vi "actuate.vi"(0 "SingleCylinderActuator in":refnum<class "SingleCylinderActuator.lvclass">, 5 "ILC in":refnum<class "ILC.lvclass">, 7 "Actuate Settings":T1, 11 "error in (no error)":errorcluster) -> (4 "SingleCylinderActuator out":refnum<class "SingleCylinderActuator.lvclass">, 6 "ILC out":refnum<class "ILC.lvclass">, 15 "error out":errorcluster)   [LabVIEW 2015, in "SingleCylinderActuator.lvclass"]
uses:
  SingleCylinderActuator.lvclass
  <userlib>/Common/ILC/ILC/ILC.lvclass
  Typedefs/Actuate Settings.ctl
  Typedefs/ControlMode.ctl
  SingleCylinderActuator.lvclass/SingleCylinderActuator.ctl
  ActuatorCylinder/IActuatorCylinder/IActuatorCylinder.lvclass
  Calculators/ForceToPressureServoVoltage/ForceToPressureServoVoltage.lvclass
  Typedefs/FAMTTypedefs.lvlib
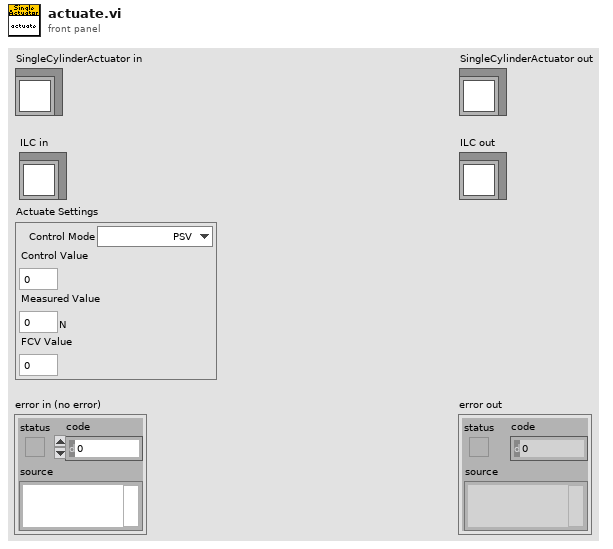
[diagram p1: front panel]
types:
  T1 = typedef "FAMTTypedefs.lvlib/Actuate Settings.ctl" = cluster{"Control Mode":T2, "Control Value":dbl, "Measured Value":dbl[unit], "FCV Value":dbl}
  T2 = typedef "FAMTTypedefs.lvlib/ControlMode.ctl" = enum16{"PSV", "FCV", "Both"}
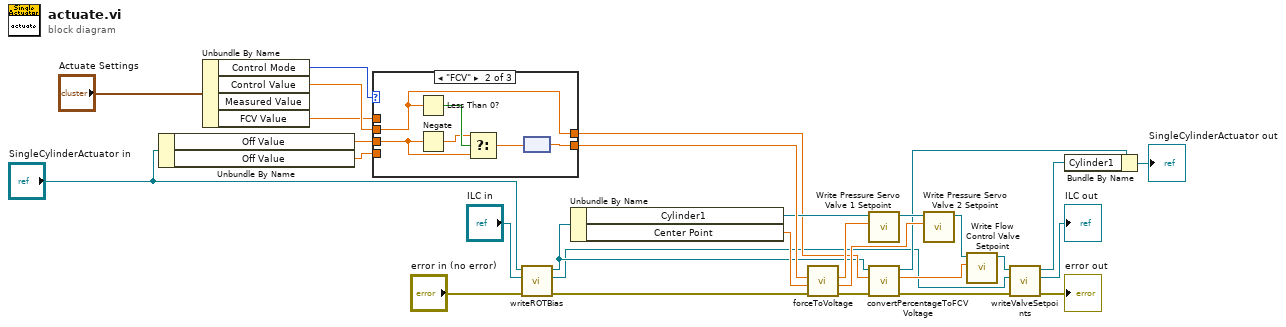
[diagram p0: block diagram]
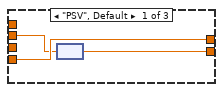
[diagram p2: hidden frame]
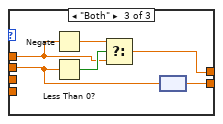
[diagram p3: hidden frame]
diagram:
  n1 = Unbundle By Name("SingleCylinderActuator in") -> ("Off Value"=w20:dbl, "Off Value"=w19:dbl)
  n2 = Unbundle By Name("Actuate Settings") -> ("Control Mode"=w25:T2, "Control Value"=w22:dbl, "FCV Value"=w21:dbl)  [unwired: 1 out]
  n3 = case shown="\"FCV\"" w25 {
    tunnel: w22 -> [w31 w37 w40]
    tunnel: w21 -> [_ _ w42]
    tunnel: w20 -> [_ w33 _]
    tunnel: w19 -> [w32 _ _]
    tunnel: [w32 w37 w41] -> w4
    tunnel: [w30 w38 w39] -> w18
    frame "PSV", Default {
      n4 = node(w31) -> (w30:dbl[unit])
    }
    frame "FCV" {
      n5 = Less Than 0?(x=w37) -> (x < 0?=w35:bool)
      n6 = Negate(x=w33) -> (-x=w34:dbl)
      n7 = Select(t=w34, s=w35, f=w33) -> (s? t:f=w36:dbl)
      n8 = node(w36) -> (w38:dbl[unit])
    }
    frame "Both" {
      n9 = Negate(x=w42) -> (-x=w43:dbl)
      n10 = Less Than 0?(x=w40) -> (x < 0?=w44:bool)
      n11 = Select(t=w43, s=w44, f=w42) -> (s? t:f=w41:dbl)
      n12 = node(w40) -> (w39:dbl[unit])
    }
  }
  n13 = call "writeROTBias.vi"("error in (no error)"="error in (no error)", "ILC in"="ILC in", "SingleCylinderActuator in"="SingleCylinderActuator in") -> ("error out"=w11:errorcluster, "ILC out"=w1:refnum<class "ILC.lvclass">, "SingleCylinderActuator out"=w3:refnum<class "SingleCylinderActuator.lvclass">)  [unwired: 6 in]
  n14 = Unbundle By Name(w3) -> ("Cylinder1"=w5:refnum<class "IActuatorCylinder.lvclass">, "Center Point"=w16:dbl[unit])
  n15 = call "forceToVoltage.vi"("error in (no error)"=w11, "Center Point"=w16, "Force"=w18) -> ("error out"=w10:errorcluster, "Voltage 2"=w23:dbl[unit], "Voltage 1"=w24:dbl[unit])  [unwired: 5 in, 1 out]
  n16 = call-dynamic "Write Pressure Servo Valve 1 Setpoint.vi"("Pressure Servo Valve 1 Setpoint"=w24, "IActuatorCylinder in"=w5) -> ("IActuatorCylinder out"=w14:refnum<class "IActuatorCylinder.lvclass">)  [unwired: 9 in]
  n17 = call "convertPercentageToFCVVoltage.vi"("error in (no error)"=w10, "Percentage"=w4, "SingleCylinderActuator in"=w3) -> ("error out"=w9:errorcluster, "Voltage"=w26:dbl, "SingleCylinderActuator out"=w2:refnum<class "SingleCylinderActuator.lvclass">)  [unwired: 6 in]
  n18 = call-dynamic "Write Pressure Servo Valve 2 Setpoint.vi"("Pressure Servo Valve 2 Setpoint"=w23, "IActuatorCylinder in"=w14) -> ("IActuatorCylinder out"=w15:refnum<class "IActuatorCylinder.lvclass">)  [unwired: 9 in]
  n19 = call-dynamic "Write Flow Control Valve Setpoint.vi"("Flow Control Valve Setpoint"=w26, "IActuatorCylinder in"=w15) -> ("IActuatorCylinder out"=w13:refnum<class "IActuatorCylinder.lvclass">)  [unwired: 9 in]
  n20 = call-dynamic "writeValveSetpoints.vi"("error in (no error)"=w9, "ILC in"=w1, "IActuatorCylinder in"=w13) -> ("error out"=→"error out":errorcluster, "ILC out"=→"ILC out":refnum<class "ILC.lvclass">, "IActuatorCylinder out"=w6:refnum<class "IActuatorCylinder.lvclass">)  [unwired: 6 in]
  n21 = Bundle By Name(cluster=w2, "Cylinder1"=w6) -> (→"SingleCylinderActuator out":refnum<class "SingleCylinderActuator.lvclass">)
